vi "tcs_acceptCommand_stopMotion.vi"(8 "error in (no error)":errorcluster, 11 "command_stopMotion_Ctl":T1) -> (0 "error out":errorcluster, 2 "function return":i32, 3 "command_stopMotion_Ctl out":T1)   [LabVIEW 2016, in "SALLV_tcs.lvlib"]
doc: "int tcs_shm_acceptCommand_stopMotionLV(tcs_command_stopMotionLV *command_stopMotion_Ctl );"
uses:
  SALLV_tcs.lvlib
  DataTypes/command_stopMotion.ctl
  SALLV_tcs.so
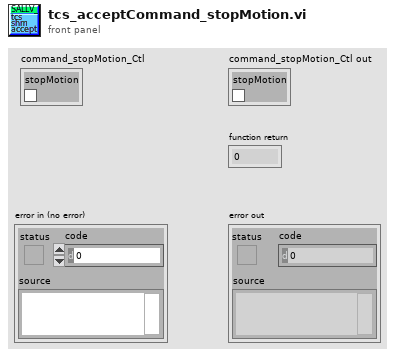
[diagram p1: front panel]
types:
  T1 = typedef "SALLV_tcs.lvlib/command_stopMotion.ctl" = cluster{"stopMotion":bool}
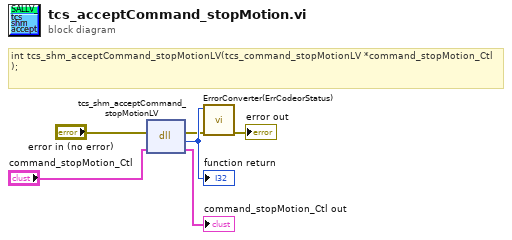
[diagram p0: block diagram]
diagram:
  # "int tcs_shm_acceptCommand_stopMotionLV(tcs_command_stopMotionLV *command_stopMotion_Ctl );"
  n1 = dll-call lib="home/andres/Desktop/SALLV_tcs/SALLV_tcs.*" fn="tcs_shm_acceptCommand_stopMotionLV"(error in="error in (no error)", "command_stopMotion_Ctl"="command_stopMotion_Ctl") -> (error out=w2:errorcluster, w6:i32, "command_stopMotion_Ctl"=→"command_stopMotion_Ctl out":T1)  [unwired: 2 in, 1 out]
  "function return" <- w6
  n2 = call "ErrorConverter(ErrCodeorStatus).vi"("error in (no error)"=w2, "error code"=w6) -> ("error out"=→"error out":errorcluster)  [unwired: 9 in]
